vi "RS485_Loopback.vi"(8 "error in (no error)":errorcluster, 10 "Parameters":string, 11 "reference in":refnum<class "Test_Flux_Capacitor.lvclass">) -> (0 "error out":errorcluster, 2 "Result":bool, 3 "reference out":refnum<class "Test_Flux_Capacitor.lvclass">)   [LabVIEW 2022 SP3, in "Test_Flux_Capacitor.lvlib" / "Test_Flux_Capacitor.lvclass"]
uses:
  Test_Flux_Capacitor.lvclass
  ParameterTypes/485_Loopback.ctl
  <vilib>/JDP Science/JSONtext/JSONtext.lvlib
panel:
  in  "Parameter_Type":T1
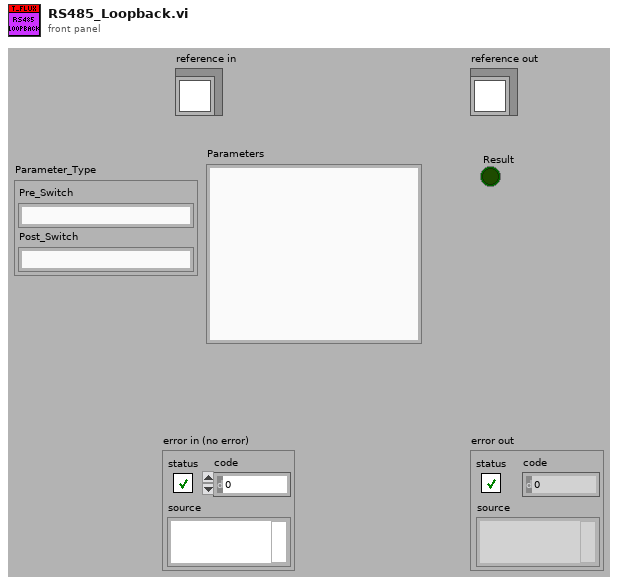
[diagram p1: front panel]
types:
  T1 = typedef "Test_Flux_Capacitor.lvlib/Test_Flux_Capacitor.lvclass/485_Loopback.ctl" = cluster{"Pre_Switch":string, "Post_Switch":string}
  T2 = typedef "Test_Flux_Capacitor.lvlib/Test_Flux_Capacitor.lvclass/ObjectAttributes.ctl" = cluster{"Config":T3, "DMM":refnum<class "DMM_Keysight_34980A.lvclass">, "LCR":refnum<class "LCR_BK891.lvclass">, "PSU":refnum<class "PSU_Base.lvclass">, "Switch_Manager":refnum<class "SwitchBase.lvclass">, "FRAM":string, "Flux_Capacitor":refnum<class "Flux_Capacitor.lvclass">, "Frequency_Counter":refnum<class "Frequency_Counter_Base.lvclass">, "JTAG":refnum<class "JTAG_Base.lvclass">}
  T3 = typedef "Test_Flux_Capacitor.lvlib/Test_Flux_Capacitor.lvclass/Config.ctl" = cluster{"default":string}
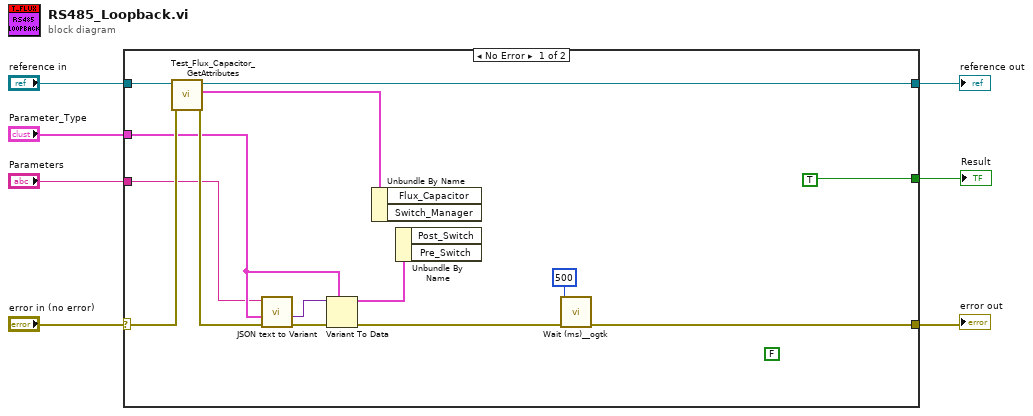
[diagram p0: block diagram]
diagram:
  n1 = case shown="No Error" "error in (no error)" {
    selector: "error in (no error)" -> [w21 w23]
    tunnel: [w9 w23] -> w6
    tunnel: [w17 w22] -> w4
    tunnel: "reference in" -> [w20 w22]
    tunnel: "Parameters" -> [w12 _]
    tunnel: "Parameter_Type" -> [w13 _]
    tunnel: [TRUE ("Connect") _] -> w1
    frame No Error {
      (unwired) FALSE ("Connect")
      n2 = call "Test_Flux_Capacitor_GetAttributes.vi"("error in (no error)"=w21, "reference in"=w20) -> ("error out"=w15:errorcluster, "Data"=w19:T2, "reference out"=w17:refnum<class "Test_Flux_Capacitor.lvclass">)  [unwired: 6 in, 1 out]
      n3 = call <vilib>:"JSON text to Variant.vi"("error in (no error)"=w15, "Data Type"=w13, "JSON"=w12) -> ("error out"=w14:errorcluster, "Variant out"=w11:variant)  [unwired: 7 in]
      n4 = Variant To Data(error in=w14, type=w13, Variant=w11) -> (data=w18:T1, error out=w10:errorcluster)
      n5 = Unbundle By Name(w19) -> ()  [unwired: 2 out]
      n6 = Unbundle By Name(w18) -> ()  [unwired: 2 out]
      n7 = call <userlib>:"Wait (ms)__ogtk.vi"("error in (no error)"=w10, "milliseconds to wait"=u32 500) -> ("error out"=w9:errorcluster)  [unwired: 8 in, 1 out]
    }
    frame Error {
    }
  }
  "Result" <- w1
  "error out" <- w6
  "reference out" <- w4
